vi "Reset Test Time.vi"(10 "Run Queue":set{string}(c389), 11 "Result Model In":refnum<class "Result Model.lvclass">) -> (3 "Result Model Out":refnum<class "Result Model.lvclass">)   [LabVIEW 2020, in "Result Model.lvclass"]
uses:
  Result Model.lvclass
  Result Model.lvclass/Result Model.ctl
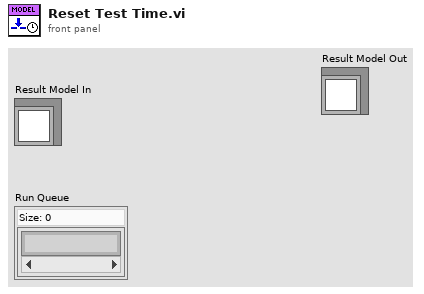
[diagram p1: front panel]
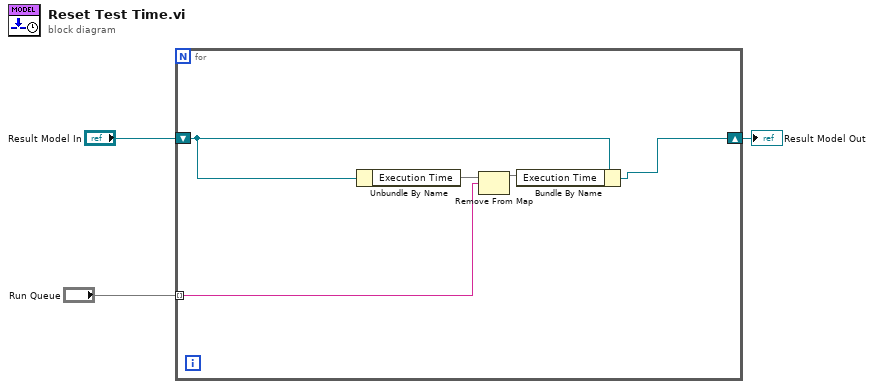
[diagram p0: block diagram]
diagram:
  n1 = for {
    tunnel: "Run Queue" -> [w8] mode=indexing
    shift-right: [w4] -> w1
    shift-left: "Result Model In" -> [w5]
    n2 = Unbundle By Name(w5) -> ("Execution Time"=w7:map{string, dbl})
    n3 = Remove From Map(10:w8, 11:w7) -> (3:w6:map{string, dbl})  [unwired: 2 out]
    n4 = Bundle By Name(cluster=w5, "Execution Time"=w6) -> (w4:refnum<class "Result Model.lvclass">)
  }
  "Result Model Out" <- w1
